vi "StartDevices.vi"(0 "Bool Refnum":refnum<vi>, 3 "Bool Refnum 2":refnum<vi>, 4 "Bool Refnum 3":refnum<vi>, 6 "error out":errorcluster, 7 "Bool Refnum 4":refnum<vi>, 12 "Bool Refnum 8":refnum<vi>, 13 "Bool Refnum 5":refnum<vi>, 15 "Bool Refnum 6":refnum<vi>, 25 "Bool Refnum 7":refnum<vi>) -> (20 "Array":cluster{"FN":T1, "Data":variant}[](array[cluster]), 24 "error out 2":errorcluster)   [LabVIEW 2011]
uses:
  Utilities/controls/ctlSeqFNs_Main.ctl
  Variables/GlobalGetCamerasOnOff.vi
  Variables/GlobalGetAvantesSpectrometerOnOff.vi
  Variables/GlobalGetAOTFOnOff.vi
  Variables/GlobalGetKoherasLaserOnOff.vi
  Variables/GlobalGetHeidenhainDriftOnOff.vi
  Variables/GlobalGetPhysikalInstrumentsOnOff.vi
  Variables/GlobalGetInitialisationStatus.vi
panel:
  in  "heidenhain":bool
  in  "Andor2":bool
  in  "AOTFGet":bool
  in  "KoherasGet":bool
  in  "E710Get":bool
  in  "E517Get":bool
  in  "Avantes":bool
  in  "Andor":bool
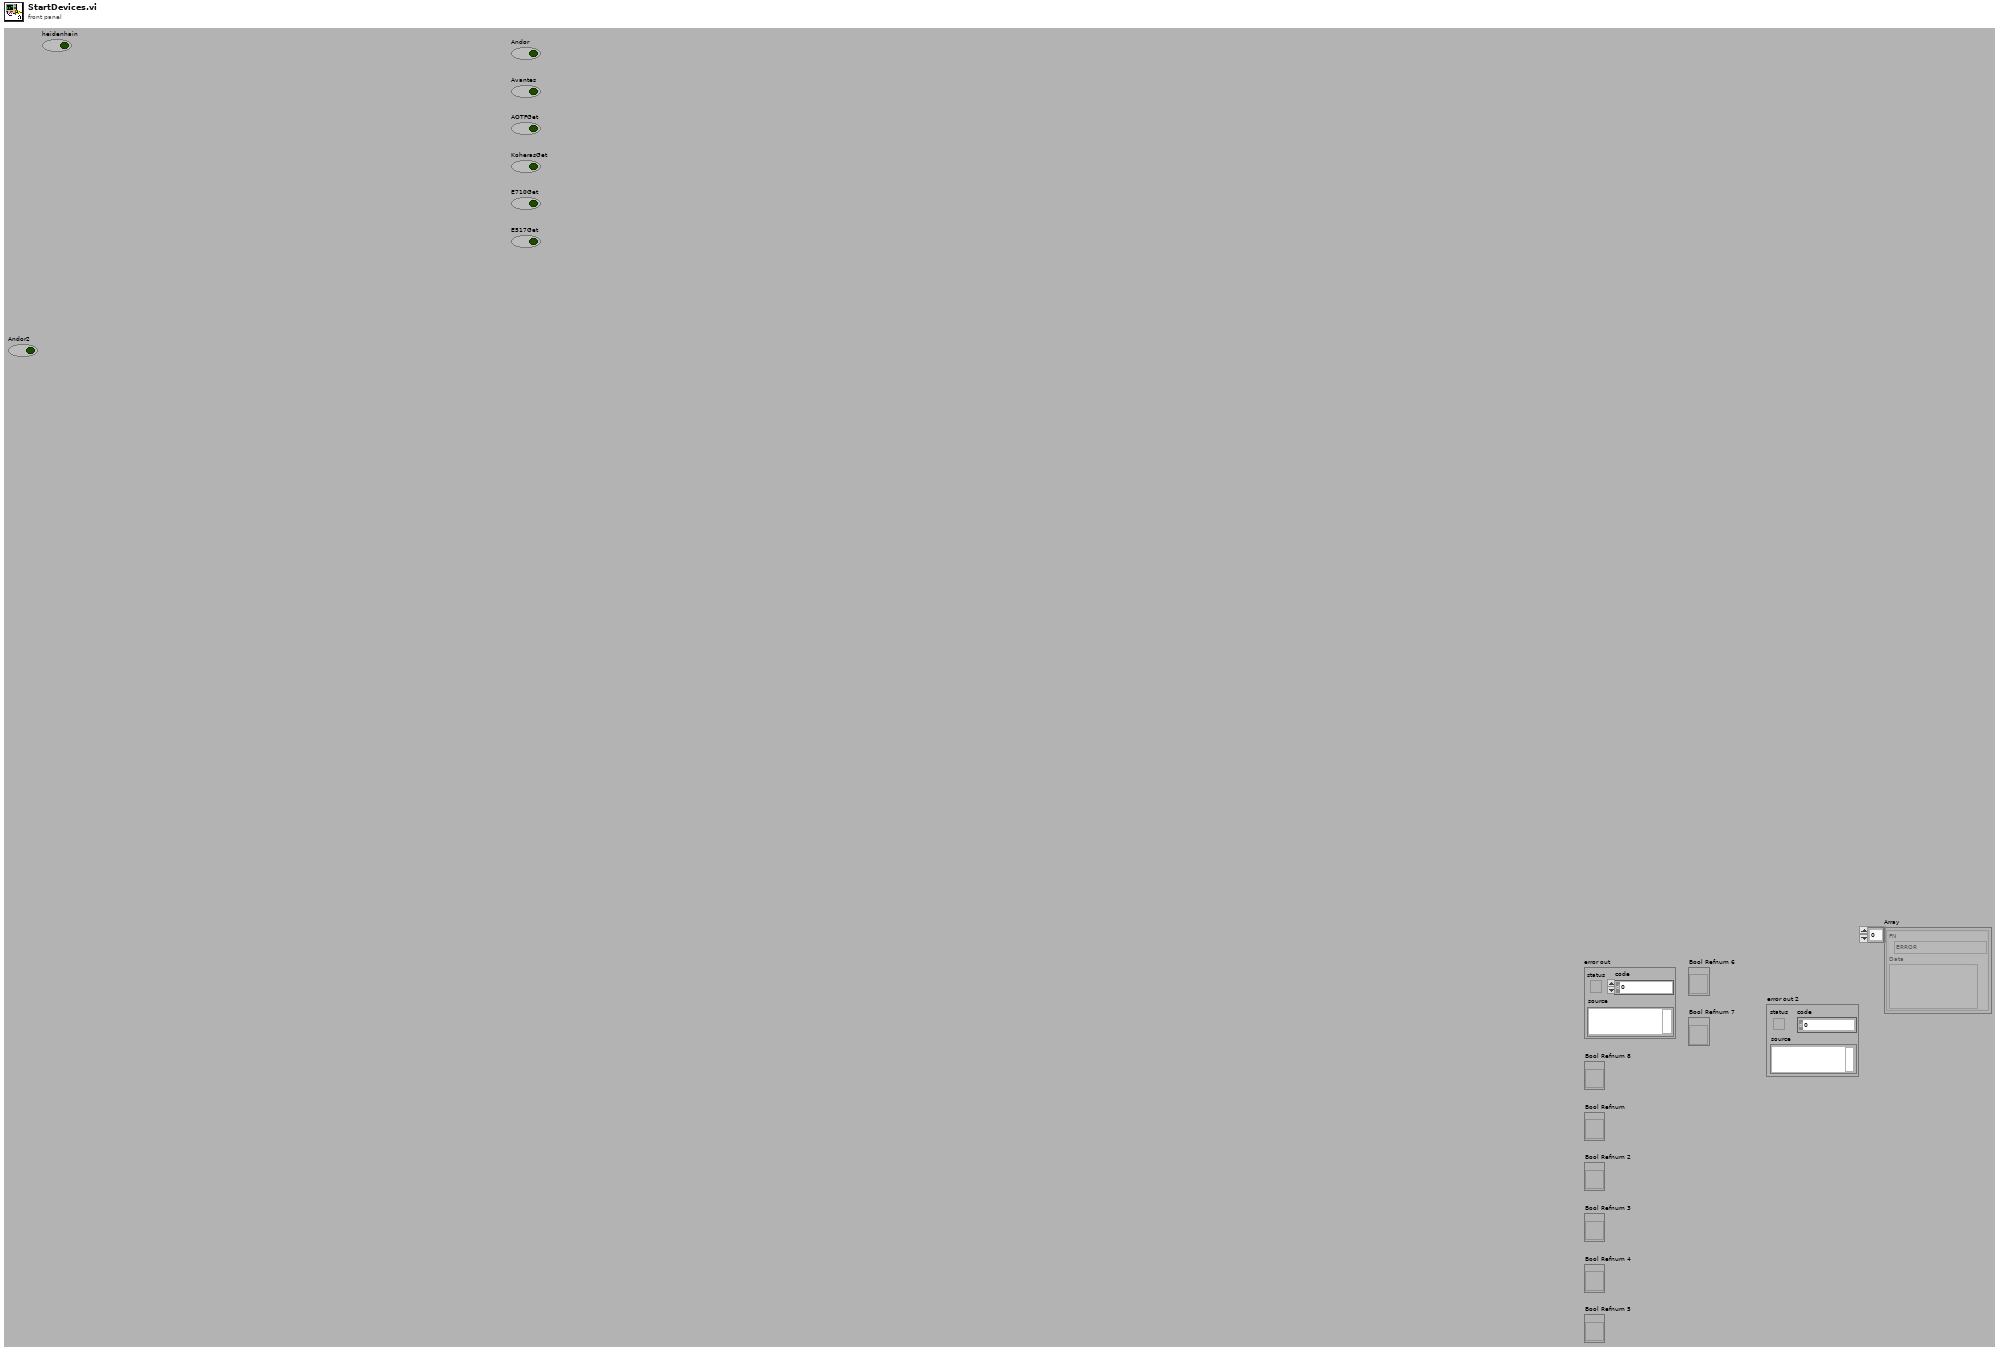
[diagram p1: front panel]
types:
  T1 = typedef "ctlSeqFNs_Main.ctl" = enum16{"ERROR", "INIT", "CONFIGURE", "MEASUREMENT", "SHUTDOWN", "IDLE", "EXIT"}
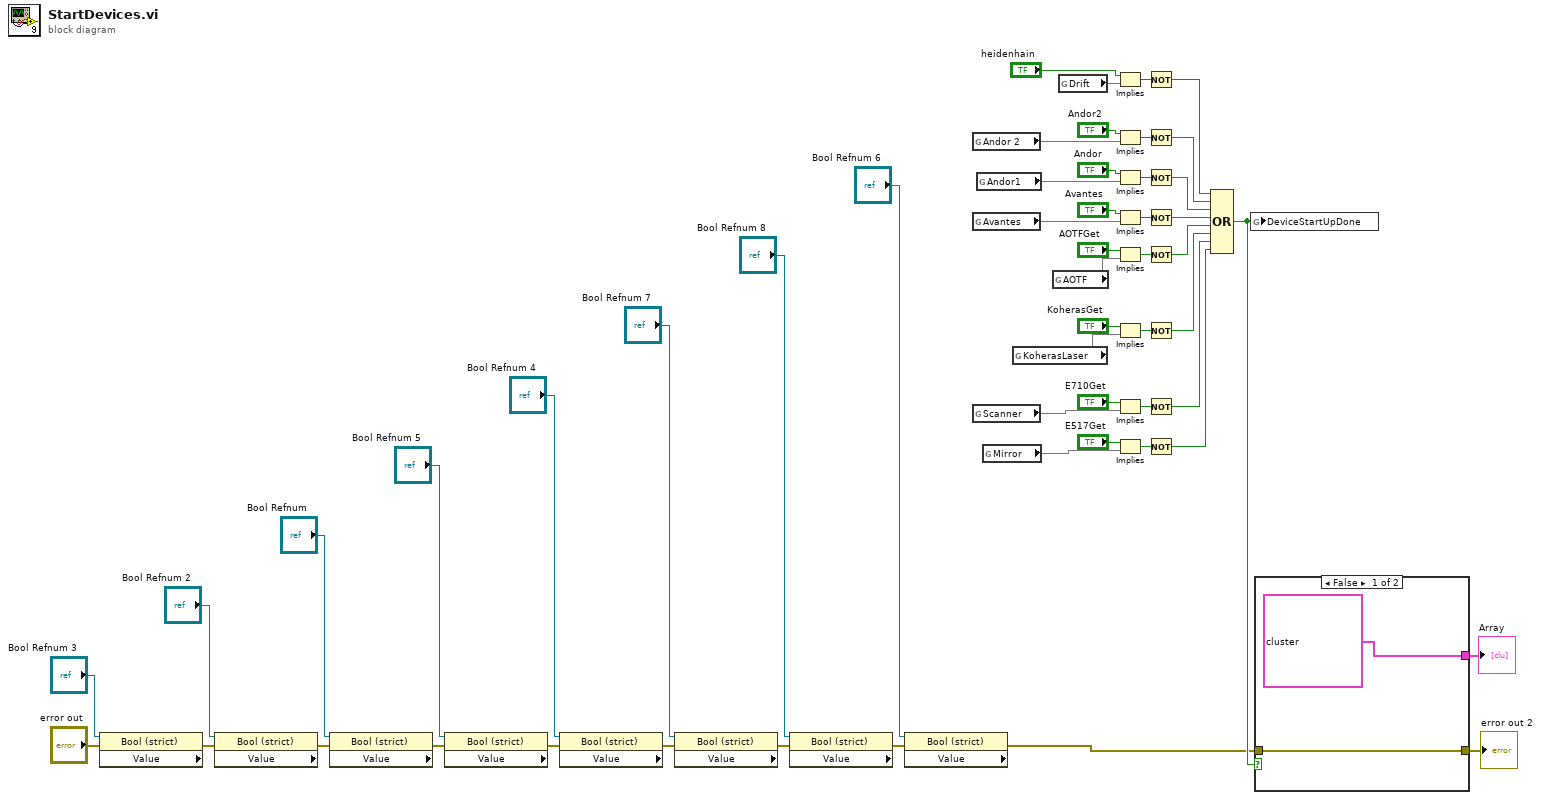
[diagram p0: block diagram]
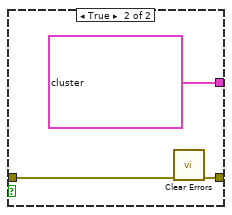
[diagram p2: hidden frame]
diagram:
  n1 = property on="Property Node" class="Bool (strict)"(reference="Bool Refnum 3", error in="error out") -> (error out=w51:errorcluster, "Value"=w46:bool)  [unwired: 1 out]
  n2 = property on="Property Node" class="Bool (strict)"(reference="Bool Refnum 2", error in=w51) -> (error out=w52:errorcluster, "Value"=w49:bool)  [unwired: 1 out]
  n3 = property on="Property Node" class="Bool (strict)"(reference="Bool Refnum", error in=w52) -> (error out=w53:errorcluster, "Value"=w48:bool)  [unwired: 1 out]
  n4 = property on="Property Node" class="Bool (strict)"(reference="Bool Refnum 5", error in=w53) -> (error out=w54:errorcluster, "Value"=w45:bool)  [unwired: 1 out]
  n5 = property on="Property Node" class="Bool (strict)"(reference="Bool Refnum 4", error in=w54) -> (error out=w56:errorcluster, "Value"=w47:bool)  [unwired: 1 out]
  n6 = property on="Property Node" class="Bool (strict)"(reference="Bool Refnum 7", error in=w56) -> (error out=w57:errorcluster, "Value"=w60:bool)  [unwired: 1 out]
  n7 = property on="Property Node" class="Bool (strict)"(reference="Bool Refnum 8", error in=w57) -> (error out=w58:errorcluster, "Value"=w59:bool)  [unwired: 1 out]
  n8 = property on="Property Node" class="Bool (strict)"(reference="Bool Refnum 6", error in=w58) -> (error out=w1:errorcluster, "Value"=w55:bool)  [unwired: 1 out]
  n9 = global read "GlobalGetCamerasOnOff.vi" "Andor 2"() -> (w9)
  n10 = global read "GlobalGetAvantesSpectrometerOnOff.vi" "Avantes"() -> (w8)
  n11 = global read "GlobalGetPhysikalInstrumentsOnOff.vi" "Scanner"() -> (w5)
  n12 = global read "GlobalGetCamerasOnOff.vi" "Andor1"() -> (w10)
  n13 = global read "GlobalGetPhysikalInstrumentsOnOff.vi" "Mirror"() -> (w4)
  n14 = global read "GlobalGetKoherasLaserOnOff.vi" "KoherasLaser"() -> (w6)
  n15 = global read "GlobalGetAOTFOnOff.vi" "AOTF"() -> (w7)
  n16 = global read "GlobalGetHeidenhainDriftOnOff.vi" "Drift"() -> (w3)
  n17 = Implies(1:w3, 2:"heidenhain") -> (0:w13:bool)
  n18 = Implies(1:w9, 2:"Andor2") -> (0:w16:bool)
  n19 = Implies(1:w10, 2:"Andor") -> (0:w23:bool)
  n20 = Implies(1:w8, 2:"Avantes") -> (0:w24:bool)
  n21 = Implies(1:w7, 2:"AOTFGet") -> (0:w25:bool)
  n22 = Implies(1:w6, 2:"KoherasGet") -> (0:w26:bool)
  n23 = Implies(1:w5, 2:"E710Get") -> (0:w27:bool)
  n24 = Implies(1:w4, 2:"E517Get") -> (0:w28:bool)
  n25 = Not(x=w13) -> (.not. x?=w12:bool)
  n26 = Not(x=w16) -> (.not. x?=w14:bool)
  n27 = Not(x=w23) -> (.not. x?=w29:bool)
  n28 = Not(x=w24) -> (.not. x?=w30:bool)
  n29 = Not(x=w25) -> (.not. x?=w31:bool)
  n30 = Not(x=w26) -> (.not. x?=w32:bool)
  n31 = Not(x=w27) -> (.not. x?=w33:bool)
  n32 = Not(x=w28) -> (.not. x?=w34:bool)
  n33 = Compound Arithmetic op=OR(w12, w14, w29, w30, w31, w32, w33, w34) -> (w2:bool)
  n34 = global write "GlobalGetInitialisationStatus.vi" "DeviceStartUpDone"(w2) -> ()
  n35 = case shown="False" w2 {
    tunnel: w1 -> [w62 w64]
    tunnel: [w62 w65] -> w36
    tunnel: [cluster{"FN":T1, "Data":variant}[] [{"FN"=enum."IDLE", "Data"=variant}, {"FN"=enum."INIT", "Data"=variant}] cluster{"FN":T1, "Data":variant}[] [{"FN"=enum."IDLE", "Data"=variant}, {"FN"=enum."CONFIGURE", "Data"=variant}]] -> w35
    frame False {
    }
    frame True {
      n36 = call <vilib>:"Clear Errors.vi"("error in (no error)"=w64) -> ("error out"=w65:errorcluster)  [unwired: 6 in]
    }
  }
  "error out 2" <- w36
  "Array" <- w35
